vi "Open Meas File V5.vi"() -> ()   [LabVIEW 2015]
panel:
  in  "byte order":T1(ring)=enum."little-endian"
  out "NoOfWords":i32
  out "lo(x)":dbl[][](graph)
  in  "count":i32=2147483647
  in  "Open File":bool
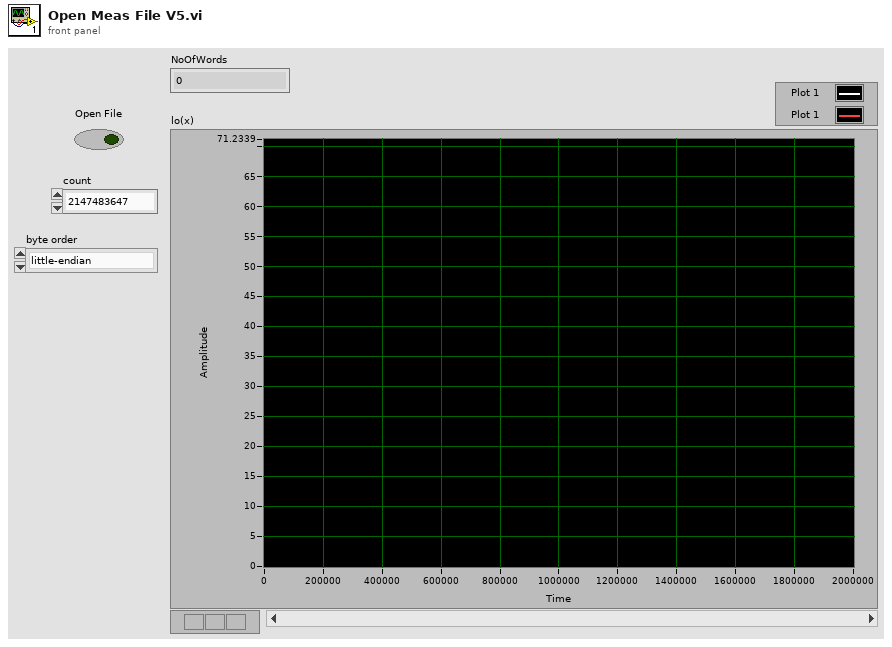
[diagram p1: front panel]
types:
  T1 = enum16{"big-endian, network order", "native, host order", "little-endian"}
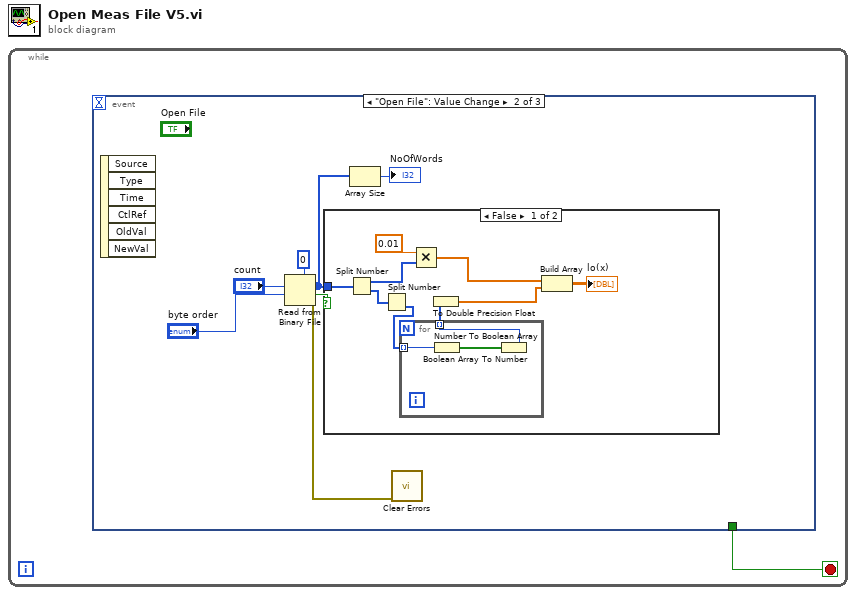
[diagram p0: block diagram]
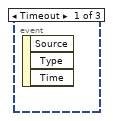
[diagram p2: hidden frame]
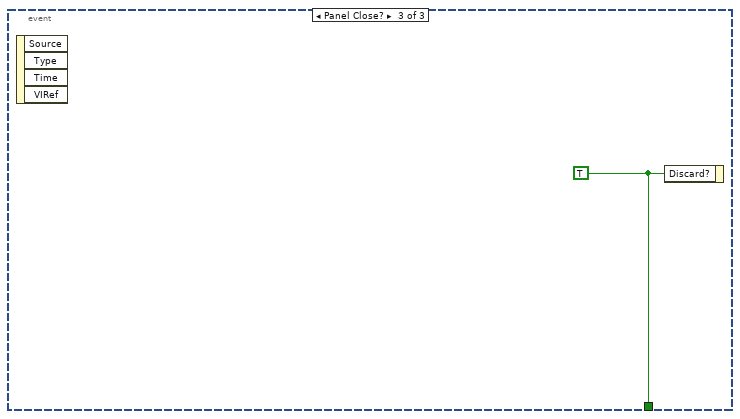
[diagram p4: hidden frame]
diagram:
  n1 = while {
    stop <- w1 stop-if-true
    n2 = event shown="[1] \"Open File\": Value Change" {
      selector: _ -> [_ _ _]
      dyn-events: _ -> [_ _ _]
      timeout: _ -> [_ _ _]
      tunnel: [_ _ w21] -> w1
      event Timeout {
        n3 = event-data() -> ()  [unwired: 1 in, 3 out]
      }
      event "Open File": Value Change {
        n4 = event-data() -> ()  [unwired: 1 in, 6 out]
        n5 = Read from Binary File(5:u64 0, 9:"byte order", 10:"count") -> (0:w5:errorcluster, 1:w6:bool, 2:w4:u64[])  [unwired: 3 in, 1 out]
        n6 = case shown="False" w6 {
          tunnel: w4 -> [w17 _]
          frame False {
            n7 = Split Number(x=w17) -> (hi(x)=w11:u32[], lo(x)=w14:u32[])
            n8 = Split Number(x=w14) -> (lo(x)=w13:u16[])  [unwired: 1 out]
            n9 = for {
              tunnel: w13 -> [w20] mode=indexing
              tunnel: [w19] -> w12 mode=indexing
              n10 = Number To Boolean Array(number=w20) -> (Boolean array=w18:bool[])
              n11 = Boolean Array To Number(Boolean array=w18) -> (number=w19:i32)
            }
            n12 = Multiply(x=0.01, y=w11) -> (x*y=w9:dbl[])
            n13 = To Double Precision Float(number=w12) -> (double precision float=w16:dbl[])
            n14 = Build Array(w9, w16) -> (→"lo(x)":dbl[][])
          }
          frame True {
          }
        }
        n15 = Array Size(array=w4) -> (size(s)=→"NoOfWords":i32)
        n16 = call <vilib>:"Clear Errors.vi"("error in (no error)"=w5) -> ()  [unwired: 5 in, 2 out]
      }
      event Panel Close? {
        w21 = TRUE ("Discard?")
        n17 = event-data() -> ()  [unwired: 1 in, 4 out]
        n18 = event-data("Discard?"=w21) -> ()  [unwired: 1 in, 1 out]
      }
    }
  }
